vi "test_LocationFGV_GetLocationThenReresolveLocation_LocationResolvedTwice.vi"(8 "error in":errorcluster) -> (0 "error out":errorcluster, 2 "result":string, 3 "pass":bool)   [LabVIEW 2020, in "MeasurementServerTests.lvlib" / "gRPC Utilities Tests.lvlib"]
uses:
  gRPC Utilities Tests.lvlib
  Fake Location Action.ctl
  Runtime/MeasurementLink Discovery/TypeDefs/Service Location FGV Action.ctl
  Runtime/MeasurementLink Discovery/MeasurementLink Discovery.lvlib
  Runtime/MeasurementLink Discovery Client/RPC Messages/ni_measurementlink_discovery_v1_ResolveServiceRequest.ctl
  Runtime/MeasurementLink Discovery Client/MeasurementLink Discovery Client.lvlib
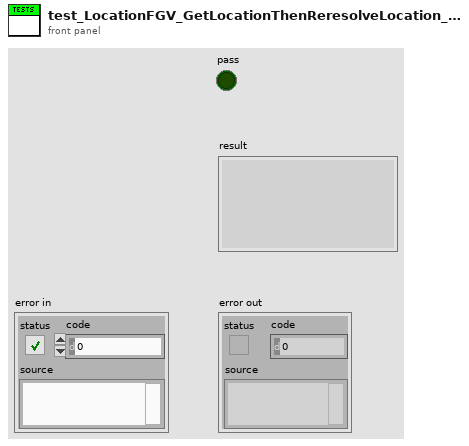
[diagram p1: front panel]
types:
  T1 = typedef "MeasurementLink Discovery.lvlib/Service Location FGV Action.ctl" = enum16{"Get Service Location", "Reresolve Service Location"}
  T2 = typedef "MeasurementLink Discovery Client.lvlib/ni_measurementlink_discovery_v1_ResolveServiceRequest.ctl" = cluster{"provided_interface":string, "service_class":string}
  T3 = typedef "MeasurementServerTests.lvlib/gRPC Utilities Tests.lvlib/Fake Location Action.ctl" = enum16{"Generate New Location", "Reset", "Error on Next Call"}
  T4 = typedef "MeasurementLink Discovery Client.lvlib/ni_measurementlink_discovery_v1_ServiceLocation.ctl" = cluster{"location":string, "insecure_port":string, "ssl_authenticated_port":string}
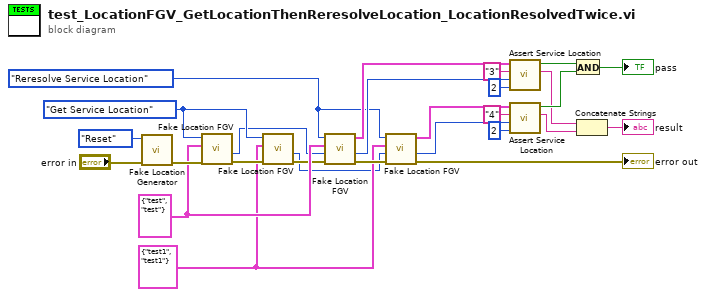
[diagram p0: block diagram]
diagram:
  w3 = Service_Location_FGV_Action."Reresolve Service Location" ("action")
  w15 = T2 {"provided_interface"="test1", "service_class"="test1"} ("resolve service request")
  w24 = T2 {"provided_interface"="test", "service_class"="test"} ("resolve service request")
  w16 = Service_Location_FGV_Action."Get Service Location" ("action")
  n1 = call "Fake Location Generator.vi"("error in"="error in", "action"=Fake_Location_Action."Reset") -> ("error out"=w26:errorcluster)  [unwired: 8 in, 1 out]
  n2 = call "Fake Location FGV.vi"("error in"=w26, "resolve service request"=w24, "action"=w16) -> ("error out"=w19:errorcluster, "unique id out"=w2:u64)  [unwired: 6 in, 1 out]
  n3 = call "Fake Location FGV.vi"("error in"=w19, "resolve service request"=w15, "action"=w16) -> ("error out"=w18:errorcluster, "unique id out"=w1:u64)  [unwired: 6 in, 1 out]
  n4 = call "Fake Location FGV.vi"("error in"=w18, "unique id in"=w2, "resolve service request"=w24, "action"=w3) -> ("error out"=w17:errorcluster, "unique id out"=w21:u64, "service location"=w23:T4)  [unwired: 5 in]
  n5 = call "Fake Location FGV.vi"("error in"=w17, "unique id in"=w1, "resolve service request"=w15, "action"=w3) -> ("error out"=→"error out":errorcluster, "unique id out"=w10:u64, "service location"=w11:T4)  [unwired: 5 in]
  n6 = call "Assert Service Location.vi"("expected unique id"=u64 2, "actual unique id"=w21, "expected service location port"="3", "actual service location"=w23) -> ("result"=w6:string, "pass"=w20:bool)  [unwired: 6 in]
  n7 = call "Assert Service Location.vi"("expected unique id"=u64 2, "actual unique id"=w10, "expected service location port"="4", "actual service location"=w11) -> ("result"=w5:string, "pass"=w7:bool)  [unwired: 6 in]
  n8 = And(x=w20, y=w7) -> (x .and. y?=→"pass":bool)
  n9 = Concatenate Strings(w6, w5) -> (→"result":string)
